vi "Lookup Or Add Variant Attribute.vi"(8 "error in (no error)":errorcluster, 9 "Initial Value":T1, 10 "Attribute Name":string, 11 "Variant in":variant) -> (0 "error out":errorcluster, 1 "Current Value":T1, 3 "Variant out":variant)   [LabVIEW 2023]
doc: "This VI adds a variant attribute if it does not already exist. It returns the current value of the attribute whether it existed before or not, without making excesssive copies of the attribute data."
uses:
  Lookup Table Data.ctl
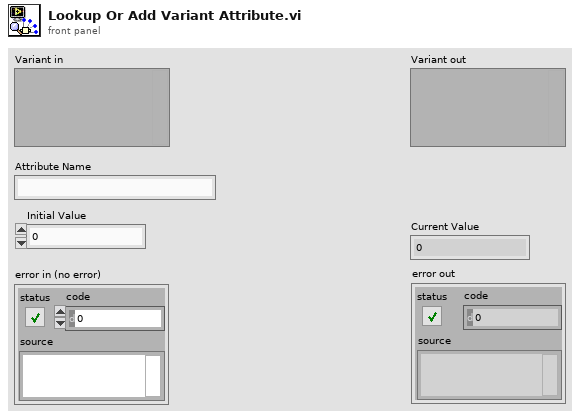
[diagram p1: front panel]
types:
  T1 = typedef "Lookup Table Data.ctl" = u32
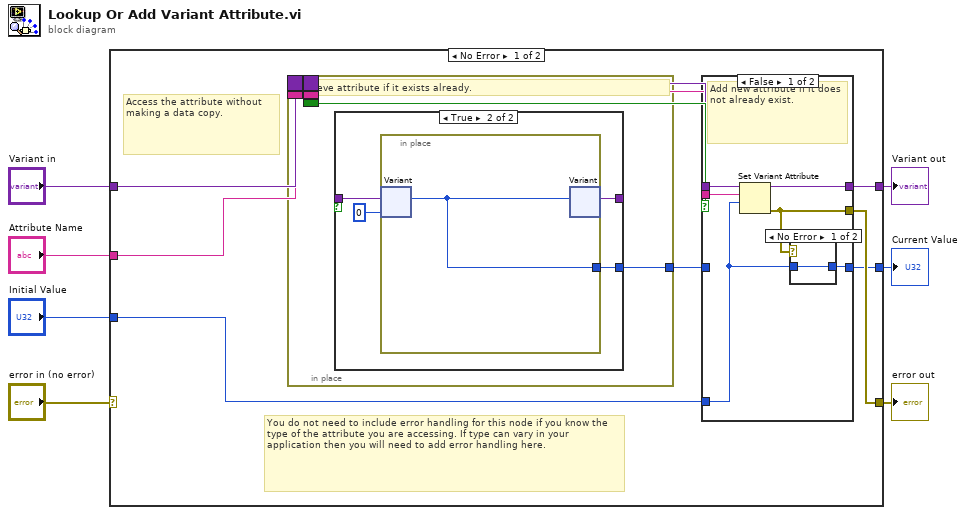
[diagram p0: block diagram]
diagram:
  n1 = case shown="No Error" "error in (no error)" {
    selector: "error in (no error)" -> [_ w37]
    tunnel: "Variant in" -> [w17 w38]
    tunnel: "Attribute Name" -> [w16 _]
    tunnel: "Initial Value" -> [w12 _]
    tunnel: [w11 w38] -> w4
    tunnel: [w10 w37] -> w2
    tunnel: [w9 _] -> w1
    frame No Error {
      # "Access the attribute without making a data copy."
      # "You do not need to include error handling for this node if you know the type of the attribute you are accessing. If type can vary in your application then you will need to add error handling here."
      n2 = in-place {
        border: w17 -> [_]
        border: w16 -> [_]
        border: [_] -> w14
        border: [_] -> w13
        border: [_] -> w15
        in-place-border: [w27] -> w8
        # "Retrieve attribute if it exists already."
        n3 = case shown="True" w30 {
          tunnel: w28 -> [w31 w35]
          tunnel: [w31 w33] -> w29
          tunnel: [_ w32] -> w27
          frame False {
          }
          frame True {
            n4 = in-place {
              in-place-border: [w36] -> w32
              n5 = in-place-variant #1(w35, T1 0 ("Increment")) -> (w36:T1)  [unwired: 1 out]
              n6 = in-place-variant #1(w36) -> (w33:variant)  [unwired: 1 out]
            }
          }
        }
      }
      n7 = case shown="False" w15 {
        tunnel: w14 -> [w23 w26]
        tunnel: w13 -> [w22 _]
        tunnel: w12 -> [w18 _]
        tunnel: [w21 w26] -> w11
        tunnel: [w20 _] -> w10
        tunnel: [w19 w25] -> w9
        tunnel: w8 -> [_ w25]
        frame False {
          # "Add new attribute if it does not already exist."
          n8 = Set Variant Attribute(Variant=w23, name=w22, value=w18) -> (Variant out=w21:variant, error out=w20:errorcluster)  [unwired: 1 in, 1 out]
          n9 = case shown="No Error" w20 {
            tunnel: [w24 _] -> w19
            tunnel: w18 -> [w24 _]
            frame No Error {
            }
            frame Error {
            }
          }
        }
        frame True {
        }
      }
    }
    frame Error {
    }
  }
  "Variant out" <- w4
  "error out" <- w2
  "Current Value" <- w1
